vi "GenerateUntriggeredStimulus.vi"(8 "error in (no error)":errorcluster, 11 "HeadorTailContinuousGWN in":refnum<class "HeadorTailContinuousGWN.lvclass">) -> (0 "error out":errorcluster, 2 "UntriggeredStimulusOut":sgl[][](array[numeric]), 3 "HeadorTailContinuousGWN out":refnum<class "HeadorTailContinuousGWN.lvclass">)   [LabVIEW 2019, in "HeadorTailContinuousGWN.lvclass"]
uses:
  HeadorTailContinuousGWN.lvclass
  D:/Github_repos/ProjectAPI/LabviewVIs/StimulusObject.lvclass
  StimulusObject.lvclass/StimulusObject.ctl
  HeadorTailContinuousGWN.lvclass/HeadorTailContinuousGWN.ctl
  ParametersGlobal.vi
  <vilib>/ptbypt/Signal Generation.llb/Gaussian White Noise PtByPt.vi
  StimulusObject.lvclass
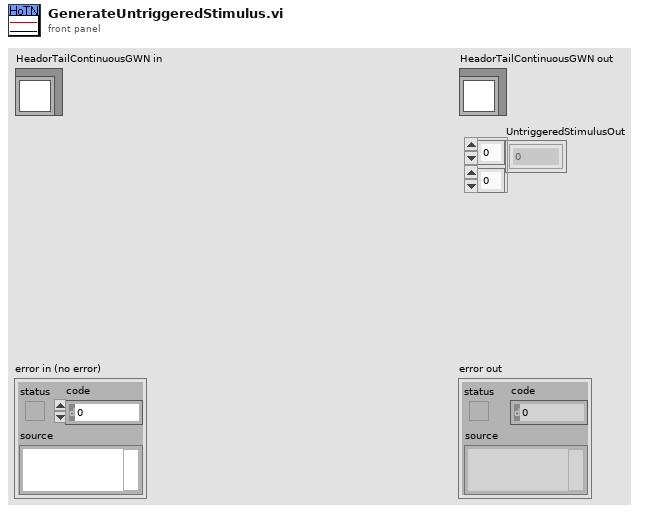
[diagram p1: front panel]
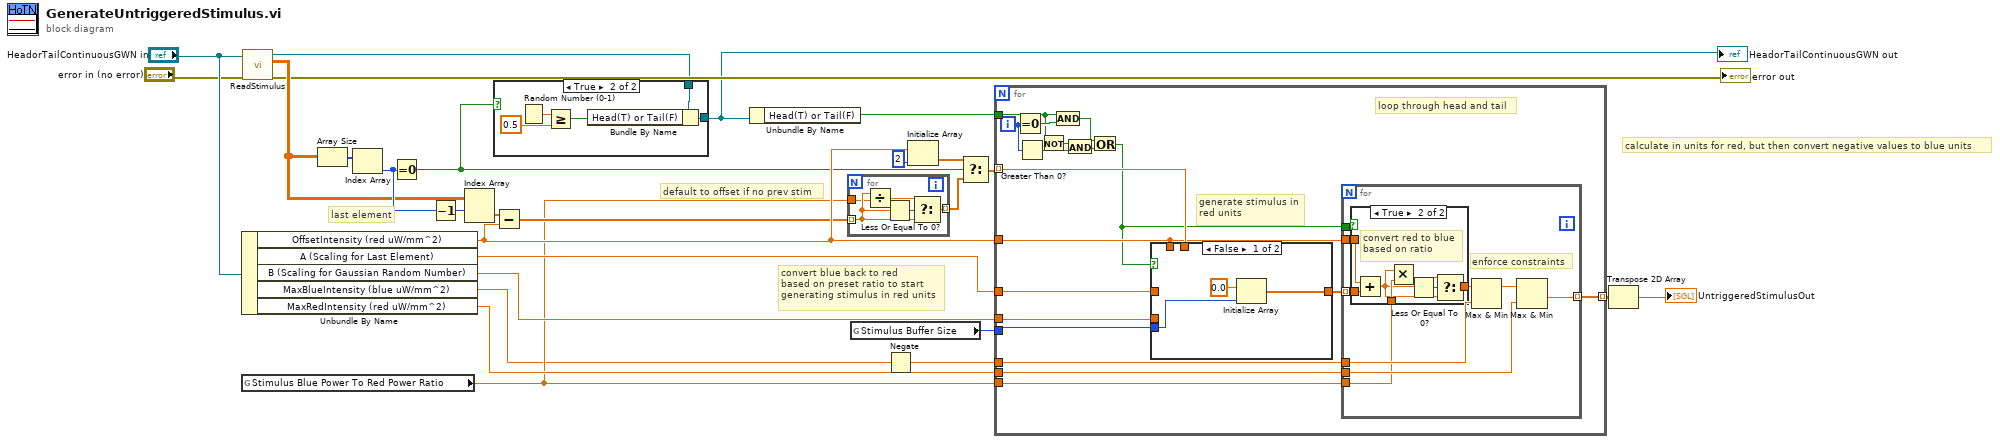
[diagram p0: block diagram]
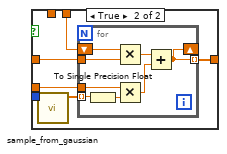
[diagram p3: hidden frame]
diagram:
  # "convert blue back to red\nbased on preset ratio to start\ngenerating stimulus in red units"
  # "calculate in units for red, but then convert negative values to blue units"
  # "default to offset if no prev stim"
  # "last element"
  n1 = Unbundle By Name("HeadorTailContinuousGWN in") -> ("OffsetIntensity (red uW/mm^2)"=w16:sgl, "A (Scaling for Last Element)"=w21:sgl, "B (Scaling for Gaussian Random Number)"=w20:sgl, "MaxBlueIntensity (blue uW/mm^2)"=w10:sgl, "MaxRedIntensity (red uW/mm^2)"=w19:sgl)
  n2 = global read "ParametersGlobal.vi" "Stimulus Blue Power To Red Power Ratio"() -> (w11:sgl)
  n3 = call "ReadStimulus.vi"("error in (no error)"="error in (no error)", "StimulusObject in"="HeadorTailContinuousGWN in") -> ("error out"=→"error out":errorcluster, "StimulusOut"=w12:sgl[][], "StimulusObject out"=w4:refnum<class "HeadorTailContinuousGWN.lvclass">)  [unwired: 7 in]
  n4 = Array Size(array=w12) -> (size(s)=w27:i32[])
  n5 = Index Array(array=w27) -> (element=w24:i32)  [unwired: 1 in]
  n6 = Equal To 0?(x=w24) -> (x = 0?=w2:bool)
  n7 = Decrement(x=w24) -> (x-1=w23:i32)
  n8 = Index Array(array=w12, index (row)=w23) -> (element=w25:sgl[])  [unwired: 1 in]
  n9 = case shown="True" w2 {
    tunnel: w4 -> [w28 w33]
    tunnel: [w28 w32] -> w3
    frame False {
    }
    frame True {
      n10 = Random Number (0-1)() -> (number: 0 to 1=w31:dbl)
      n11 = Greater Or Equal?(x=w31, y=0.5) -> (x >= y?=w29:bool)
      n12 = Bundle By Name(cluster=w33, "Head(T) or Tail(F)"=w29) -> (w32:refnum<class "HeadorTailContinuousGWN.lvclass">)
    }
  }
  "HeadorTailContinuousGWN out" <- w3
  n13 = Subtract(x=w25, y=w16) -> (x-y=w14:sgl[])
  n14 = Unbundle By Name(w3) -> ("Head(T) or Tail(F)"=w1:bool)
  n15 = for {
    tunnel: w14 -> [w35] mode=indexing
    tunnel: [w37] -> w13 mode=indexing
    tunnel: w11 -> [w34]
    n16 = Divide(x=w35, y=w34) -> (x/y=w36:sgl)
    n17 = Less Or Equal To 0?(x=w35) -> (x <= 0?=w38:bool)
    n18 = Select(t=w36, s=w38, f=w35) -> (s? t:f=w37:sgl)
  }
  n19 = global read "ParametersGlobal.vi" "Stimulus Buffer Size"() -> (w18:i32)
  n20 = Negate(x=w10) -> (-x=w9:sgl)
  n21 = Initialize Array(w16, 2 ("dimension size")) -> (w17:sgl[])
  n22 = Select(t=w17, s=w2, f=w13) -> (s? t:f=w26:sgl[])
  n23 = for {
    tunnel: w26 -> [w56] mode=indexing
    tunnel: w21 -> [w55]
    tunnel: w20 -> [w54]
    tunnel: [w53] -> w22 mode=indexing
    tunnel: w16 -> [w46]
    tunnel: w9 -> [w52]
    tunnel: w19 -> [w51]
    tunnel: w18 -> [w50]
    tunnel: w11 -> [w49]
    tunnel: w1 -> [w42]
    i -> [w45]
    # "generate stimulus in\nred units"
    # "loop through head and tail"
    n24 = Equal To 0?(x=w45) -> (x = 0?=w47:bool)
    n25 = Greater Than 0?(x=w45) -> (x > 0?=w44:bool)
    n26 = Not(x=w42) -> (.not. x?=w43:bool)
    n27 = And(x=w42, y=w47) -> (x .and. y?=w40:bool)
    n28 = And(x=w43, y=w44) -> (x .and. y?=w41:bool)
    n29 = Or(x=w40, y=w41) -> (x .or. y?=w39:bool)
    n30 = case shown="False" w39 {
      tunnel: w56 -> [_ w65]
      tunnel: w55 -> [_ w64]
      tunnel: w54 -> [_ w63]
      tunnel: w50 -> [w59 w61]
      tunnel: [w58 w60] -> w48
      tunnel: w46 -> [_ _]
      frame False {
        n31 = Initialize Array(0.0 ("element"), w59) -> (w58:dbl[])
      }
      frame True {
        n32 = call "sample_from_gaussian.vi"("Samples"=w61) -> ("Output"=w62:dbl[])  [unwired: 10 in]
        n33 = for {
          shift-right: [w66] -> _
          shift-left: w65 -> [w72]
          tunnel: w64 -> [w73]
          tunnel: w63 -> [w69]
          tunnel: w62 -> [w71] mode=indexing
          tunnel: [w66] -> w60 mode=indexing
          n34 = To Single Precision Float(number=w71) -> (single precision float=w70:sgl)
          n35 = Multiply(x=w72, y=w73) -> (x*y=w67:sgl)
          n36 = Multiply(x=w69, y=w70) -> (x*y=w68:sgl)
          n37 = Add(x=w67, y=w68) -> (x+y=w66:sgl)
        }
      }
    }
    n38 = for {
      tunnel: w48 -> [w80] mode=indexing
      tunnel: [w81] -> w53 mode=indexing
      tunnel: w46 -> [w79]
      tunnel: w52 -> [w78]
      tunnel: w51 -> [w77]
      tunnel: w49 -> [w75]
      tunnel: w39 -> [w74]
      # "enforce constraints"
      n39 = case shown="True" w74 {
        tunnel: w80 -> [w83 w90]
        tunnel: w79 -> [_ w89]
        tunnel: [w83 w86] -> w76
        tunnel: w75 -> [_ w85]
        frame False {
        }
        frame True {
          # "convert red to blue\nbased on ratio"
          n40 = Add(x=w89, y=w90) -> (x+y=w84:dbl)
          n41 = Multiply(x=w84, y=w85) -> (x*y=w87:dbl)
          n42 = Less Or Equal To 0?(x=w84) -> (x <= 0?=w88:bool)
          n43 = Select(t=w87, s=w88, f=w84) -> (s? t:f=w86:dbl)
        }
      }
      n44 = Max & Min(x=w76, y=w78) -> (max(x,y)=w82:dbl)  [unwired: 1 out]
      n45 = Max & Min(x=w82, y=w77) -> (min(x,y)=w81:dbl)  [unwired: 1 out]
    }
  }
  n46 = Transpose 2D Array(2D array=w22) -> (transposed array=→"UntriggeredStimulusOut":dbl[][])
